vi "Cross_moments_simple.vi"(0 "U":dbl[](array[numeric]) format="%.2f", 1 "W":dbl[](array[numeric]) format="%.2f", 2 "Block No":i32=1, 5 "Shift in":dbl[](array[numeric]) format="%.2f") -> (14 "Correlation":dbl format="%.2f", 19 "Shift out":dbl[](array[numeric]) format="%.2f")   [LabVIEW 2010]
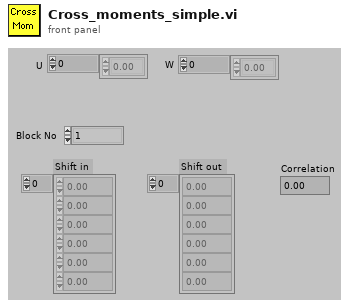
[diagram p1: front panel]
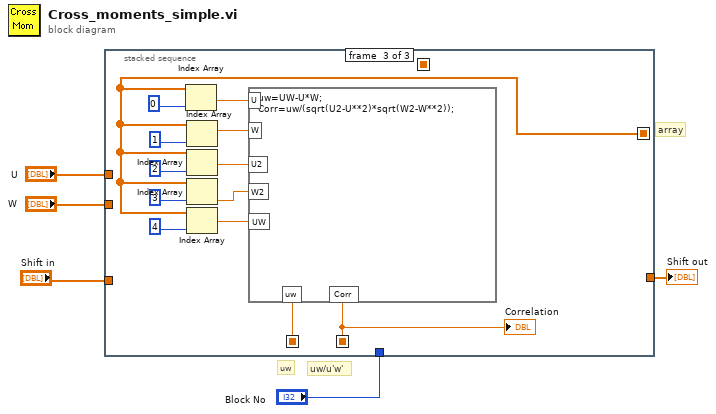
[diagram p0: block diagram]
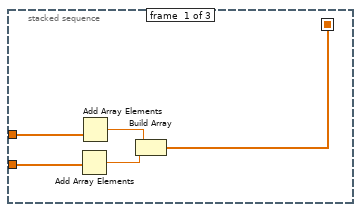
[diagram p2: hidden frame]
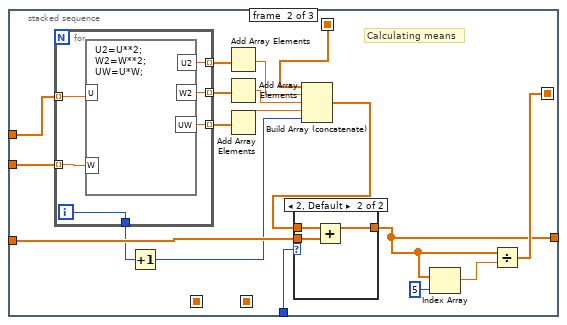
[diagram p3: hidden frame]
diagram:
  # "array"
  # "uw/u'w'"
  # "uw"
  n1 = stacked-sequence {
    seq-local: [_ _ w46] -> [_ _ _]
    seq-local: [_ _ w45] -> [_ _ _]
    seq-local: [_ w27 _] -> [_ _ w39]
    seq-local: [w6 _ _] -> [_ w11 _]
    tunnel: "U" -> [w10 w21 _]
    tunnel: [_ w13 _] -> w4
    tunnel: "Shift in" -> [_ w28 _]
    tunnel: "Block No" -> [_ w26 _]
    tunnel: "W" -> [w9 w22 _]
    frame #0 {
      n2 = Add Array Elements(numeric array=w9) -> (sum=w7:dbl)
      n3 = Add Array Elements(numeric array=w10) -> (sum=w8:dbl)
      n4 = Build Array(w8, w7) -> (w6:dbl[])
    }
    frame #1 {
      # "Calculating means"
      n5 = for {
        tunnel: w21 -> [w38] mode=indexing
        tunnel: w22 -> [w37] mode=indexing
        tunnel: [w36] -> w20 mode=indexing
        tunnel: [w35] -> w19 mode=indexing
        tunnel: [w34] -> w18 mode=indexing
        tunnel: [w33] -> w16
        i -> [w33]
        n6 = formula code="U2=U**2;\nW2=W**2;\nUW=U*W;"("U"=w38, "W"=w37) -> ("U2"=w36:dbl, "W2"=w35:dbl, "UW"=w34:dbl)
      }
      n7 = Increment(x=w16) -> (x+1=w15:i32)
      n8 = Add Array Elements(numeric array=w20) -> (sum=w17:dbl)
      n9 = Add Array Elements(numeric array=w19) -> (sum=w25:dbl)
      n10 = Add Array Elements(numeric array=w18) -> (sum=w24:dbl)
      n11 = Build Array (concatenate)(w11, w17, w25, w24, w15) -> (w23:dbl[])
      n12 = case shown="2, Default" w26 {
        tunnel: [w29 w30] -> w13
        tunnel: w28 -> [_ w32]
        tunnel: w23 -> [w29 w31]
        frame 1 {
        }
        frame 2, Default {
          n13 = Add(x=w31, y=w32) -> (x+y=w30:dbl[])
        }
      }
      n14 = Index Array(array=w13, index=5 ("Index")) -> (element=w12:dbl)
      n15 = Divide(x=w13, y=w12) -> (x/y=w27:dbl[])
    }
    frame #2 {
      n16 = Index Array(array=w39, index=0) -> (element=w44:dbl)
      n17 = Index Array(array=w39, index=1) -> (element=w43:dbl)
      n18 = Index Array(array=w39, index=2) -> (element=w42:dbl)
      n19 = Index Array(array=w39, index=3) -> (element=w41:dbl)
      n20 = Index Array(array=w39, index=4) -> (element=w40:dbl)
      n21 = formula code="uw=UW-U*W;\nCorr=uw/(sqrt(U2-U**2)*sqrt(W2-W**2));"("W"=w43, "W2"=w41, "U"=w44, "U2"=w42, "UW"=w40) -> ("uw"=w46:dbl, "Corr"=w45:dbl)
      "Correlation" <- w45
    }
  }
  "Shift out" <- w4
